vi "Is_It_Too_Short_Track_for_Subtrack-1.vi"(1 "[IN] Minimal Subtrack Length \n(Points without problems) for\nMaking Desicion":i32, 2 "[IN] Statuses of point in track":i16[](array[numeric])) -> (0 "[OUT] Points enough":bool)   [LabVIEW 2013]
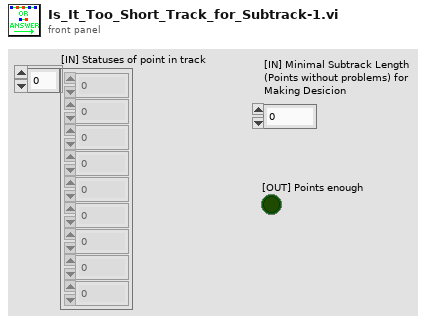
[diagram p1: front panel]
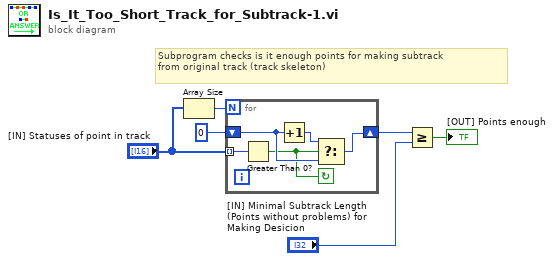
[diagram p0: block diagram]
diagram:
  # "Subprogram checks is it enough points for making subtrack\nfrom original track (track skeleton)"
  n1 = Array Size(array="[IN] Statuses of point in track") -> (size(s)=w6:i32)
  n2 = for {
    N: w6 -> [_]
    tunnel: "[IN] Statuses of point in track" -> [w11] mode=indexing
    shift-right: [w8] -> w3
    shift-left: 0 -> [w9]
    stop <- w7 continue-if-true
    n3 = Greater Than 0?(x=w11) -> (x > 0?=w7:bool)
    n4 = Increment(x=w9) -> (x+1=w10:i32)
    n5 = Select(t=w10, s=w7, f=w9) -> (s? t:f=w8:i32)
  }
  n6 = Greater Or Equal?(x=w3, y="[IN] Minimal Subtrack Length \n(Points without problems) for\nMaking Desicion") -> (x >= y?=→"[OUT] Points enough":bool)
